vi "EnQueue_Message_Single.vi"(6 "Priority Message? (F)":bool, 8 "error in (no error)":errorcluster, 9 "Message Data":variant, 10 "Message":string, 11 "Message_Queue":refnum<queue>) -> (0 "error out":errorcluster, 3 "Dup_Message_Queue":refnum<queue>)   [LabVIEW 2014]
uses:
  02_Controls/Message_Data_Ctl.ctl
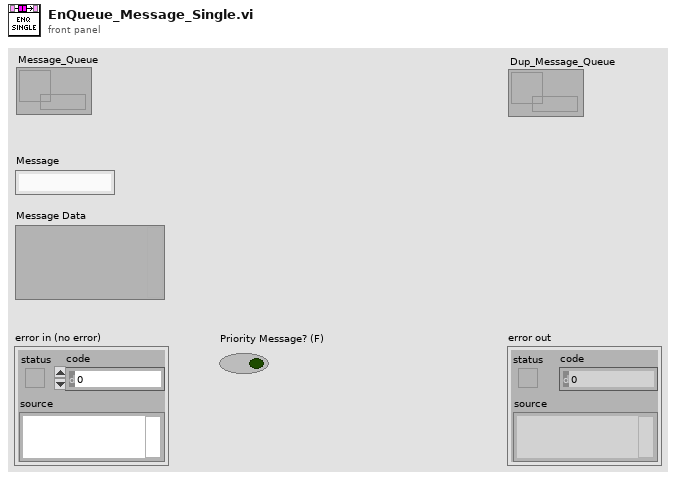
[diagram p1: front panel]
types:
  T1 = typedef "Message_Data_Ctl.ctl" = cluster{"Message":string, "Data":variant}
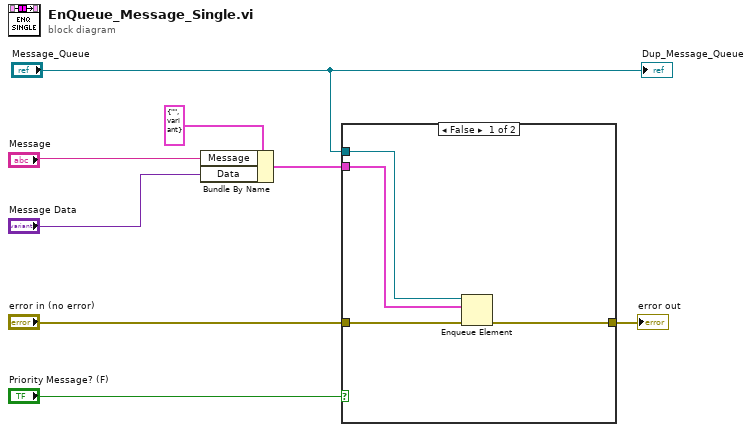
[diagram p0: block diagram]
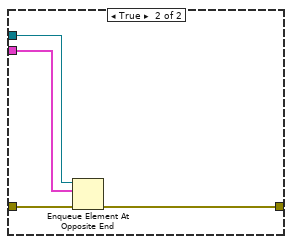
[diagram p2: hidden frame]
diagram:
  n1 = Bundle By Name(cluster=T1 {"Message"="", "Data"=variant} ("Message_Data"), "Message"="Message", "Data"="Message Data") -> (w3:T1)
  n2 = case shown="False" "Priority Message? (F)" {
    tunnel: "error in (no error)" -> [w12 w16]
    tunnel: [w11 w15] -> w4
    tunnel: "Message_Queue" -> [w10 w14]
    tunnel: w3 -> [w9 w13]
    frame False {
      n3 = Enqueue Element(queue=w10, element=w9, error in (no error)=w12) -> (error out=w11:errorcluster)  [unwired: 1 in, 2 out]
    }
    frame True {
      n4 = Enqueue Element At Opposite End(queue=w14, element=w13, error in (no error)=w16) -> (error out=w15:errorcluster)  [unwired: 1 in, 2 out]
    }
  }
  "error out" <- w4
  "Dup_Message_Queue" <- "Message_Queue"
